vi "(auto) Set Manip.vi"(5 "G_upper bound":i32, 7 "M_lower bound":i32, 8 "error in (no error)":errorcluster) -> (0 "error out":errorcluster)   [LabVIEW 2017]
uses:
  <vilib>/myRIO/Instrument Drivers/Onboard IO/PWM/typedefs/PWM Reference.ctl
  <vilib>/myRIO/Common/Instrument Driver Framework/Utilities/typedefs/myRIO Generic Hardware Reference.ctl
  <vilib>/myRIO/Common/Instrument Driver Framework/Utilities/typedefs/Hardware Version Enum.ctl
  <vilib>/myRIO/Common/Instrument Driver Framework/Utilities/typedefs/myRIO v1.0 Reference.ctl
  <vilib>/myRIO/Common/Instrument Driver Framework/Utilities/typedefs/Generic FPGA Reference.ctl
  <vilib>/myRIO/Common/Instrument Driver Framework/myRIO v1.0/PWM/typedefs/PWM Channels Enum.ctl
  <vilib>/myRIO/Instrument Drivers/Onboard IO/PWM/typedefs/PWM Configuration.ctl
  <vilib>/userdefined/High Color/nirio_resource_hc.ctl
  <vilib>/myRIO/Common/Instrument Driver Framework/myRIO v1.0/Encoder/typedefs/Encoder Configuration v1.0.ctl
  <vilib>/myRIO/Common/Instrument Driver Framework/myRIO v1.0/Encoder/typedefs/Encoder Signal Mode.ctl
  <vilib>/myRIO/Instrument Drivers/Onboard IO/Encoder/typedefs/Encoder Reference.ctl
  <vilib>/myRIO/Common/Instrument Driver Framework/myRIO v1.0/Encoder/typedefs/Encoder Channels Enum.ctl
  <vilib>/myRIO/Instrument Drivers/Onboard IO/DIO/typedefs/DIO Reference.ctl
  <vilib>/myRIO/Common/Instrument Driver Framework/myRIO v1.0/DIO/typedefs/DIO Channels List.ctl
  <vilib>/myRIO/Common/Instrument Driver Framework/myRIO v1.0/DIO/typedefs/DIO Channels Enum.ctl
  <vilib>/myRIO/Common/Instrument Driver Framework/Utilities/vis/Is FPGA Ref Available.vi
  <vilib>/myRIO/Common/Instrument Driver Framework/myRIO v1.0/PWM/vis/myRIO v1.1 Open PWM.vi
  <vilib>/myRIO/Instrument Drivers/Onboard IO/PWM/vis/Set Duty Cycle and Frequency.vi
  <vilib>/myRIO/Common/Instrument Driver Framework/myRIO v1.0/Encoder/vis/myRIO v1.1 Open Encoder.vi
  <vilib>/myRIO/Common/Instrument Driver Framework/myRIO v1.0/DIO/vis/myRIO v1.1 Open DIO.vi
  <vilib>/myRIO/Instrument Drivers/Onboard IO/DIO/vis/Write.vi
  <vilib>/myRIO/Common/Instrument Driver Framework/Utilities/vis/Validate Channels.vi
  <vilib>/myRIO/Common/Instrument Driver Framework/myRIO v1.0/PWM/vis/myRIO v1.0 Reserve PWM.vi
  <vilib>/myRIO/Common/Instrument Driver Framework/myRIO v1.0/Encoder/vis/myRIO v1.0 Reserve Encoder.vi
  <vilib>/myRIO/Common/Instrument Driver Framework/myRIO v1.0/DIO/vis/myRIO v1.0 Reserve DIO.vi
  <vilib>/myRIO/Common/Instrument Driver Framework/myRIO v1.0/Encoder/vis/myRIO v1.0 Close Encoder.vi
  <vilib>/myRIO/Common/Instrument Driver Framework/myRIO v1.0/PWM/vis/myRIO v1.0 Build MUX Configuration PWM.vi
  <vilib>/myRIO/Common/Instrument Driver Framework/myRIO v1.0/Resource Manager/vis/myRIO v1.0 Reserve Channel List.vi
  <vilib>/myRIO/Common/Instrument Driver Framework/myRIO v1.0/Encoder/vis/myRIO v1.0 Build MUX Configuration Encoder.vi
  <vilib>/myRIO/Common/Instrument Driver Framework/myRIO v1.0/DIO/vis/myRIO v1.0 Build MUX Configuration DIO.vi
  <vilib>/myRIO/Common/Instrument Driver Framework/myRIO v1.0/Encoder/vis/myRIO v1.0 Unreserve Encoder.vi
  <vilib>/myRIO/Common/Instrument Driver Framework/myRIO v1.0/Resource Manager/vis/myRIO v1.0 Create Configuration List.vi
  <vilib>/myRIO/Common/Instrument Driver Framework/myRIO v1.0/Resource Manager/vis/myRIO v1.0 Reserve Channel.vi
  <vilib>/myRIO/Common/Instrument Driver Framework/myRIO v1.0/Resource Manager/vis/myRIO v1.0 Unreserve Channel.vi
  <vilib>/myRIO/Common/Instrument Driver Framework/myRIO v1.0/Resource Manager/vis/myRIO v1.0 Unreserve Channel List.vi
  <vilib>/myRIO/Common/Instrument Driver Framework/myRIO v1.0/Resource Manager/vis/myRIO v1.0 Build Mutex Name.vi
  <vilib>/Utility/VariantDataType/GetNumericInfo.vi
  <vilib>/Utility/error.llb/Error Cluster From Error Code.vi
  <vilib>/myRIO/Common/Instrument Driver Framework/myRIO v1.0/myRIO v1.1 Open.vi
  <vilib>/myRIO/Common/Instrument Driver Framework/Utilities/vis/IO Manager.vi
  <vilib>/myRIO/Common/Instrument Driver Framework/Utilities/vis/Configuration Manager.vi
  <vilib>/myRIO/Common/Instrument Driver Framework/myRIO v1.0/Resource Manager/vis/myRIO v1.0 Configure IO.vi
  <vilib>/myRIO/Common/Instrument Driver Framework/myRIO v1.0/myRIO v1.0 Close.vi
  <vilib>/myRIO/Common/Instrument Driver Framework/myRIO v1.0/Encoder/vis/myRIO v1.0 Configure Encoder.vi
  <vilib>/myRIO/Common/Instrument Driver Framework/myRIO v1.0/Encoder/vis/myRIO v1.0 Reset Encoder.vi
  <vilib>/myRIO/Common/Instrument Driver Framework/myRIO v1.0/PWM/vis/myRIO v1.0 Write PWM.vi
  <vilib>/myRIO/Common/Instrument Driver Framework/myRIO v1.0/Encoder/vis/myRIO v1.0 Read Encoder.vi
  <vilib>/myRIO/Common/Instrument Driver Framework/myRIO v1.0/DIO/vis/myRIO v1.0 Write DIO.vi
  <vilib>/myRIO/Common/Instrument Driver Framework/myRIO v1.0/Encoder/vis/myRIO v1.0 Shutdown Encoder.vi
  <vilib>/myRIO/Instrument Drivers/Onboard IO/Encoder/vis/myRIO Encoder Open.xnode
  <vilib>/myRIO/Express VI/Onboard IO/PWM/PWM Express VI.xnode
  <vilib>/myRIO/Instrument Drivers/Onboard IO/PWM/vis/myRIO PWM Open.xnode
  <vilib>/myRIO/Express VI/Onboard IO/DO/DO Express VI.xnode
  <vilib>/myRIO/Instrument Drivers/Onboard IO/DIO/vis/myRIO DIO Open.xnode
  <vilib>/myRIO/Instrument Drivers/Onboard IO/Encoder/Encoder.lvlib
  <vilib>/myRIO/Instrument Drivers/Onboard IO/DIO/DIO.lvlib
  <vilib>/myRIO/Instrument Drivers/Onboard IO/PWM/PWM.lvlib
panel:
  in  "resetG?":bool
  in  "range":i32=50
  in  "G_PWM":dbl=0.4
  in  "M_PWM":dbl=0.4
  in  "resetM?":bool
  out "G enc val":i32
  out "G+":bool
  in  "stopG":bool
  in  "G- (B/DIO7 (Pin 25))":bool
  in  "G+ (B/DIO13 (Pin 26))":bool
  out "ArrG_enc_val":i32[](array[numeric])
  out "M enc val":i32
  in  "stopM":bool
  out "M+":bool
  in  "offset":i32=50
  in  "frames to pass":i32=100
  in  "iterations control":i32=10
  in  "M+ (B/DIO5 (Pin 21))":bool
  in  "M- (B/DIO6 (Pin 23))":bool
  in  "offset for Extra Stop":i32=100
  out "ArrM_enc_val":i32[](array[numeric])
  in  "def it":i32=100
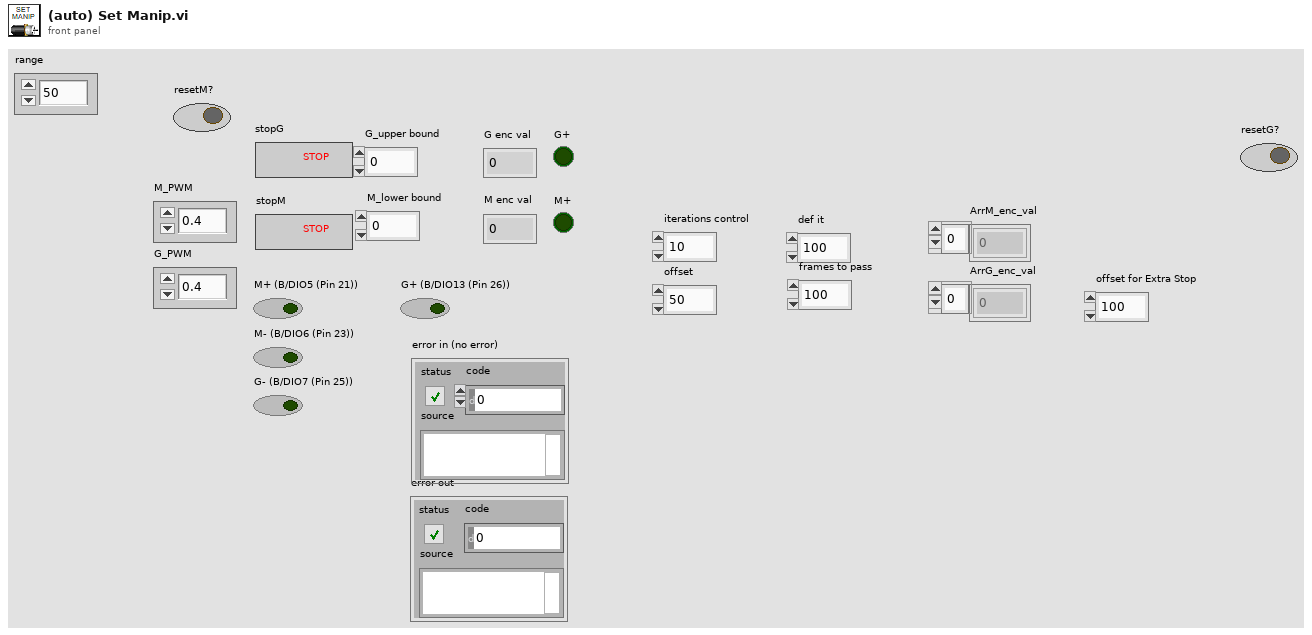
[diagram p1: front panel]
types:
  T1 = typedef "PWM.lvlib/PWM Reference.ctl" = cluster{"myRIO Reference":T2, "PWM Channels Enum":T6, "PWM Configuration":T7}
  T2 = typedef "myRIO Generic Hardware Reference.ctl" = cluster{"myRIO Model":T3, "myRIO Hardware Reference":T4}
  T3 = typedef "Hardware Version Enum.ctl" = enum16{"Unknown", "myRIO-1900", "myRIO-1950", "roboRIO", "NI ELVIS RIO CM"}
  T4 = typedef "myRIO v1.0 Reference.ctl" = cluster{"Generic FPGA Reference":T5, "Allow multiple opens":bool}
  T5 = typedef "Generic FPGA Reference.ctl" = refnum<k20>
  T6 = typedef "PWM Channels Enum.ctl" = enum16{"Not Connected", "C/PWM0", "C/PWM1", "A/PWM0", "A/PWM1", "A/PWM2", "B/PWM0", "B/PWM1", "B/PWM2", "PWM/PWM0", "PWM/PWM1", "PWM/PWM2", "PWM/PWM3", "PWM/PWM4", "PWM/PWM5", "PWM/PWM6", "PWM/PWM7", "PWM/PWM8", "PWM/PWM9"}
  T7 = typedef "PWM.lvlib/PWM Configuration.ctl" = cluster{"Frequency":dbl, "Duty Cycle":dbl}
  T8 = typedef "nirio_resource_hc.ctl" = tag
  T9 = typedef "DIO.lvlib/DIO Reference.ctl" = cluster{"myRIO Reference":T2, "DIO Channels List":T10}
  T10 = typedef "DIO Channels List.ctl" = T11[]
  T11 = typedef "DIO Channels Enum.ctl" = enum16{"Not Connected", "C/DIO0", "C/DIO1", "C/DIO2", "C/DIO3", "C/DIO4", "C/DIO5", "C/DIO6", "C/DIO7", "A/DIO0", "A/DIO1", "A/DIO2", "A/DIO3", "A/DIO4", "A/DIO5", "A/DIO6", "A/DIO7", "A/DIO8", "A/DIO9", "A/DIO10", "A/DIO11", "A/DIO12", "A/DIO13", "A/DIO14", "A/DIO15", "B/DIO0", "B/DIO1", "B/DIO2", "B/DIO3", "B/DIO4", "B/DIO5", "B/DIO6", "B/DIO7", "B/DIO8", "B/DIO9", "B/DIO10", "B/DIO11", "B/DIO12", "B/DIO13", "B/DIO14", "B/DIO15", "LED0", "LED1", "LED2", "LED3", "Button0", "DIO/DIO0", "DIO/DIO1", "DIO/DIO2", "DIO/DIO3", "DIO/DIO4", "DIO/DIO5", "DIO/DIO6", "DIO/DIO7", "DIO/DIO8", "DIO/DIO9", "SPI/CS0", "SPI/CS1", "SPI/CS2", "SPI/CS3", "LED RADIO (Green)", "LED RADIO (Red)", "LED COMM (Green)", "LED COMM (Red)", "LED MODE (Green)", "LED MODE (Red)"}
  T12 = typedef "Encoder.lvlib/Encoder Reference.ctl" = cluster{"myRIO Reference":T2, "Encoder Channels Enum":T13}
  T13 = typedef "Encoder Channels Enum.ctl" = enum16{"Not Connected", "C/ENC0", "C/ENC1", "A/ENC", "B/ENC", "DIO/ENC0", "DIO/ENC1", "DIO/ENC2", "DIO/ENC3", "DIO/ENC4"}
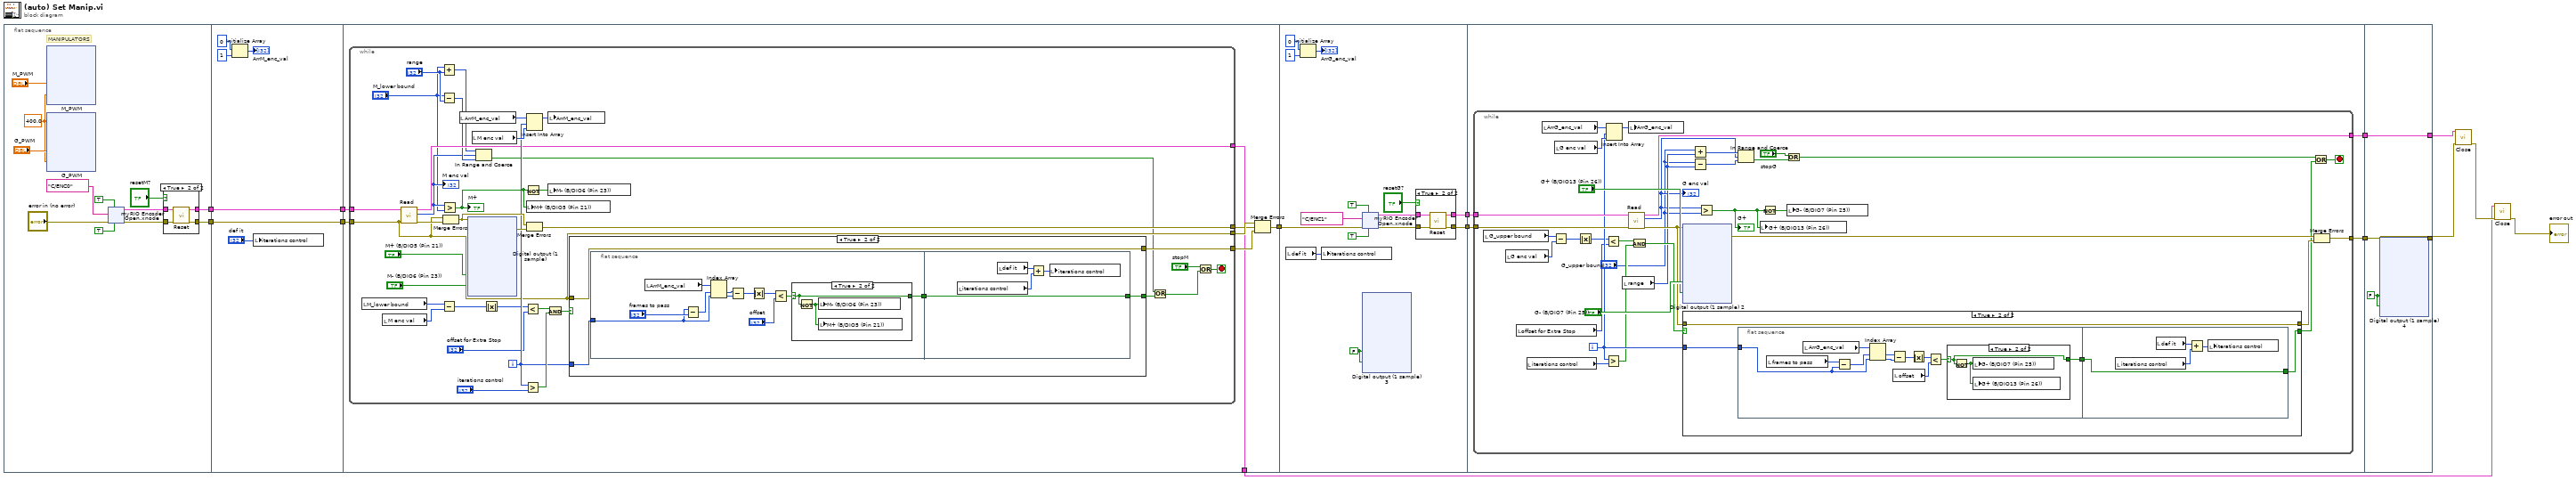
[diagram p0: block diagram]
diagram:
  n1 = flat-sequence {
    tunnel: [w20] -> w10
    tunnel: [w19] -> w9
    tunnel: [w124] -> w14
    tunnel: [w125] -> w13
    tunnel: w10 -> [w124]
    tunnel: w9 -> [w125]
    tunnel: w14 -> [w136]
    tunnel: w13 -> [w133]
    tunnel: [w131] -> w3
    tunnel: [w130] -> w8
    tunnel: [w234] -> w12
    tunnel: [w235] -> w11
    tunnel: w8 -> [w233]
    tunnel: w12 -> [w312]
    tunnel: w11 -> [w311]
    tunnel: [w310] -> w2
    tunnel: [w309] -> w1
    tunnel: [w408] -> w7
    tunnel: [w409] -> w6
    tunnel: w2 -> [w409]
    tunnel: w1 -> [w408]
    frame #0 {
      w15 = 400.0 ("Frequency [Hz]")
      # "MANIPULATORS"
      n2 = xnode "M_PWM"("Duty Cycle"="M_PWM", "Frequency [Hz]"=w15) -> ()  [unwired: 1 in, 1 out]
      n3 = xnode "G_PWM"("Duty Cycle"="G_PWM", "Frequency [Hz]"=w15) -> ()  [unwired: 1 in, 1 out]
      n4 = xnode "myRIO Encoder Open.xnode"("error in (no error)"="error in (no error)", "Allow multiple opens?"=TRUE, "Channel Name"=tag "C/ENC0", "Start Counter"=TRUE) -> ("error out"=w21:errorcluster, "Encoder Ref Out"=w22:T12)  [unwired: 1 in]
      n5 = case shown="True" "resetM?" {
        tunnel: w22 -> [w98 w102]
        tunnel: w21 -> [w97 w101]
        tunnel: [w97 w100] -> w20
        tunnel: [w98 w99] -> w19
        frame False {
        }
        frame True {
          n6 = call <vilib>:"Reset.vi"("error in (no error)"=w101, "Encoder Ref In"=w102) -> ("error out"=w100:errorcluster, "Encoder Ref Out"=w99:T12)  [unwired: 8 in]
        }
      }
    }
    frame #1 {
      n7 = Initialize Array(0 ("dimension size"), 1 ("dimension size")) -> (→"ArrM_enc_val":i32[])
      n8 = local write "iterations control"("def it") -> ()
    }
    frame #2 {
      n9 = while {
        tunnel: w136 -> [w158]
        tunnel: [w158] -> w135
        tunnel: [w171] -> w134
        tunnel: w133 -> [w170]
        tunnel: [w157] -> w132
        tunnel: [w146] -> w131
        i -> [w159]
        stop <- w156 stop-if-true
        n10 = local read "M_lower bound"() -> (w151:i32)
        n11 = local read "M enc val"() -> (w152:i32)
        n12 = call <vilib>:"Read.vi"("error in (no error)"=w158, "Encoder Ref In"=w170) -> ("error out"=w169:errorcluster, "Counter Value"=w138:i32, "Encoder Ref Out"=w146:T12)  [unwired: 5 in, 2 out]
        "M enc val" <- w138
        n13 = Add(x="M_lower bound", y="range") -> (x+y=w142:i32)
        n14 = Subtract(x="M_lower bound", y="range") -> (x-y=w143:i32)
        n15 = Subtract(x=w151, y=w152) -> (x-y=w149:i32)
        n16 = Greater?(x=w138, y="M_lower bound") -> (0:w145:bool)
        "M+" <- w145
        n17 = Merge Errors(w158, w169) -> (w166:errorcluster)
        n18 = local read "ArrM_enc_val"() -> (w162:i32[])
        n19 = xnode "Digital output (1 sample)"("M+ (B/DIO5 (Pin 21))"="M+ (B/DIO5 (Pin 21))", "M- (B/DIO6 (Pin 23))"="M- (B/DIO6 (Pin 23))", "error in (no error)"=w166) -> ("error out"=w167:errorcluster)
        n20 = local read "M enc val"() -> (w160:i32)
        n21 = In Range and Coerce(upper limit=w142, x=w138, lower limit=w143) -> (In Range?=w139:bool)  [unwired: 1 out]
        n22 = Absolute Value(x=w149) -> (abs(x)=w147:i32)
        n23 = Less?(x=w147, y="offset for Extra Stop") -> (x < y?=w150:bool)
        n24 = Greater?(x=w159, y="iterations control") -> (0:w164:bool)
        n25 = Not(x=w145) -> (.not. x?=w144:bool)
        n26 = Insert Into Array(array=w162, index=w159, new element=w160) -> (w161:i32[])
        n27 = local write "M+ (B/DIO5 (Pin 21))"(w145) -> ()
        n28 = Merge Errors(w166, w167) -> (w171:errorcluster)
        n29 = And(x=w150, y=w164) -> (x .and. y?=w153:bool)
        n30 = local write "ArrM_enc_val"(w161) -> ()
        n31 = local write "M- (B/DIO6 (Pin 23))"(w144) -> ()
        n32 = case shown="True" w153 {
          selector: w153 -> [w172 _]
          tunnel: w159 -> [_ w177]
          tunnel: w158 -> [w173 w176]
          tunnel: [w173 w176] -> w157
          tunnel: [w172 w174] -> w165
          frame False {
          }
          frame True {
            n33 = flat-sequence {
              tunnel: w177 -> [w185]
              tunnel: [w178] -> w175
              tunnel: [w192] -> w174
              tunnel: w175 -> [w192]
              frame #0 {
                n34 = local read "ArrM_enc_val"() -> (w188:i32[])
                n35 = Subtract(x=w185, y="frames to pass") -> (x-y=w186:i32)
                n36 = Index Array(array=w188, index #1=w186, index #2=w185) -> (element #1=w184:i32, element #2=w183:i32)
                n37 = Subtract(x=w184, y=w183) -> (x-y=w182:i32)
                n38 = Absolute Value(x=w182) -> (abs(x)=w181:i32)
                n39 = Less?(x=w181, y="offset") -> (x < y?=w179:bool)
                n40 = case shown="True" w179 {
                  selector: w179 -> [w189 w190]
                  tunnel: [w189 w190] -> w178
                  frame False {
                  }
                  frame True {
                    n41 = Not(x=w190) -> (.not. x?=w191:bool)
                    n42 = local write "M- (B/DIO6 (Pin 23))"(w191) -> ()
                    n43 = local write "M+ (B/DIO5 (Pin 21))"(w191) -> ()
                  }
                }
              }
              frame #1 {
                n44 = local read "iterations control"() -> (w195:i32)
                n45 = local read "def it"() -> (w193:i32)
                n46 = Add(x=w193, y=w195) -> (x+y=w194:i32)
                n47 = local write "iterations control"(w194) -> ()
              }
            }
          }
        }
        n48 = Or(x=w139, y=w165) -> (x .or. y?=w140:bool)
        n49 = Or(x="stopM", y=w140) -> (x .or. y?=w156:bool)
      }
      n50 = Merge Errors(w135, w134, w132) -> (w130:errorcluster)
    }
    frame #3 {
      w232 = FALSE ("M+ (B/DIO5 (Pin 21))")
      n51 = local read "def it"() -> (w243:i32)
      n52 = Initialize Array(0 ("dimension size"), 1 ("dimension size")) -> (→"ArrG_enc_val":i32[])
      n53 = local write "iterations control"(w243) -> ()
      n54 = xnode "myRIO Encoder Open.xnode"("error in (no error)"=w233, "Allow multiple opens?"=TRUE, "Channel Name"=tag "C/ENC1", "Start Counter"=TRUE) -> ("error out"=w237:errorcluster, "Encoder Ref Out"=w238:T12)  [unwired: 1 in]
      n55 = xnode "Digital output (1 sample) 3"("M+ (B/DIO5 (Pin 21))"=w232, "M- (B/DIO6 (Pin 23))"=w232) -> ()  [unwired: 1 in, 1 out]
      n56 = case shown="True" "resetG?" {
        tunnel: w238 -> [w283 w287]
        tunnel: w237 -> [w282 w286]
        tunnel: [w282 w285] -> w234
        tunnel: [w283 w284] -> w235
        frame False {
        }
        frame True {
          n57 = call <vilib>:"Reset.vi"("error in (no error)"=w286, "Encoder Ref In"=w287) -> ("error out"=w285:errorcluster, "Encoder Ref Out"=w284:T12)  [unwired: 8 in]
        }
      }
    }
    frame #4 {
      n58 = while {
        tunnel: w312 -> [w346]
        tunnel: [w334] -> w310
        tunnel: w311 -> [w343]
        tunnel: [w321] -> w309
        i -> [w336]
        stop <- w331 stop-if-true
        n59 = local read "G_upper bound"() -> (w325:i32)
        n60 = local read "G enc val"() -> (w326:i32)
        n61 = local read "offset for Extra Stop"() -> (w324:i32)
        n62 = local read "iterations control"() -> (w338:i32)
        n63 = local read "ArrG_enc_val"() -> (w339:i32[])
        n64 = Subtract(x=w325, y=w326) -> (x-y=w327:i32)
        n65 = local read "G enc val"() -> (w340:i32)
        n66 = Absolute Value(x=w327) -> (abs(x)=w322:i32)
        n67 = Less?(x=w322, y=w324) -> (x < y?=w323:bool)
        n68 = Greater?(x=w336, y=w338) -> (0:w332:bool)
        n69 = Insert Into Array(array=w339, index=w336, new element=w340) -> (w337:i32[])
        n70 = local read "range"() -> (w318:i32)
        n71 = local write "ArrG_enc_val"(w337) -> ()
        n72 = call <vilib>:"Read.vi"("error in (no error)"=w346, "Encoder Ref In"=w343) -> ("error out"=w335:errorcluster, "Counter Value"=w316:i32, "Encoder Ref Out"=w321:T12)  [unwired: 5 in, 2 out]
        "G enc val" <- w316
        n73 = And(x=w323, y=w332) -> (x .and. y?=w328:bool)
        n74 = xnode "Digital output (1 sample) 2"("G- (B/DIO7 (Pin 25))"="G- (B/DIO7 (Pin 25))", "G+ (B/DIO13 (Pin 26))"="G+ (B/DIO13 (Pin 26))", "error in (no error)"=w335) -> ("error out"=w344:errorcluster)
        n75 = case shown="True" w328 {
          selector: w328 -> [w347 _]
          tunnel: w336 -> [_ w352]
          tunnel: w335 -> [w348 w351]
          tunnel: [w348 w351] -> w333
          tunnel: [w347 w350] -> w329
          frame False {
          }
          frame True {
            n76 = flat-sequence {
              tunnel: w352 -> [w358]
              tunnel: [w353] -> w349
              tunnel: [w367] -> w350
              tunnel: w349 -> [w367]
              frame #0 {
                n77 = local read "frames to pass"() -> (w356:i32)
                n78 = local read "ArrG_enc_val"() -> (w363:i32[])
                n79 = Subtract(x=w356, y=w358) -> (x-y=w357:i32)
                n80 = Index Array(array=w363, index #1=w357, index #2=w358) -> (element #1=w360:i32, element #2=w355:i32)
                n81 = Subtract(x=w360, y=w355) -> (x-y=w362:i32)
                n82 = local read "offset"() -> (w354:i32)
                n83 = Absolute Value(x=w362) -> (abs(x)=w361:i32)
                n84 = Less?(x=w361, y=w354) -> (x < y?=w359:bool)
                n85 = case shown="True" w359 {
                  selector: w359 -> [w364 w365]
                  tunnel: [w364 w365] -> w353
                  frame False {
                  }
                  frame True {
                    n86 = Not(x=w365) -> (.not. x?=w366:bool)
                    n87 = local write "G- (B/DIO7 (Pin 25))"(w366) -> ()
                    n88 = local write "G+ (B/DIO13 (Pin 26))"(w366) -> ()
                  }
                }
              }
              frame #1 {
                n89 = local read "iterations control"() -> (w369:i32)
                n90 = local read "def it"() -> (w368:i32)
                n91 = Add(x=w368, y=w369) -> (x+y=w370:i32)
                n92 = local write "iterations control"(w370) -> ()
              }
            }
          }
        }
        n93 = Add(x="G_upper bound", y=w318) -> (x+y=w320:i32)
        n94 = Subtract(x="G_upper bound", y=w318) -> (x-y=w319:i32)
        n95 = Greater?(x=w316, y="G_upper bound") -> (0:w313:bool)
        "G+" <- w313
        n96 = In Range and Coerce(upper limit=w320, x=w316, lower limit=w319) -> (In Range?=w317:bool)  [unwired: 1 out]
        n97 = local write "G+ (B/DIO13 (Pin 26))"(w313) -> ()
        n98 = Not(x=w313) -> (.not. x?=w314:bool)
        n99 = Or(x="stopG", y=w317) -> (x .or. y?=w330:bool)
        n100 = local write "G- (B/DIO7 (Pin 25))"(w314) -> ()
        n101 = Or(x=w330, y=w329) -> (x .or. y?=w331:bool)
        n102 = Merge Errors(w344, w333) -> (w334:errorcluster)
      }
    }
    frame #5 {
      w407 = FALSE ("G- (B/DIO7 (Pin 25))")
      n103 = xnode "Digital output (1 sample) 4"("G- (B/DIO7 (Pin 25))"=w407, "G+ (B/DIO13 (Pin 26))"=w407) -> ()  [unwired: 1 in, 1 out]
    }
  }
  n104 = call <vilib>:"Close.vi"("error in (no error)"=w6, "Encoder Ref In"=w7) -> ("error out"=w5:errorcluster)  [unwired: 9 in]
  n105 = call <vilib>:"Close.vi"("error in (no error)"=w5, "Encoder Ref In"=w3) -> ("error out"=→"error out":errorcluster)  [unwired: 9 in]
